vi "DBM_GetTimesRange.vi"(8 "error in (no error)":errorcluster, 9 "End time":timestamp, 10 "Start time":timestamp, 11 "DBManager in":refnum<class "DBManager.lvclass">) -> (0 "error out":errorcluster, 2 "Work period":T1[](array[typedef]), 3 "DBManager out":refnum<class "DBManager.lvclass">)   [LabVIEW 2015, in "DBManager.lvclass"]
uses:
  DBManager.lvclass
  WorkDay.ctl
  DBManager.lvclass/DBManager.ctl
  <vilib>/drjdpowell/SQLite Library/SQL Statement/SQL Statement.lvclass/SQL Statement.ctl
  <vilib>/drjdpowell/SQLite Library/SQL Statement/Column I64.vi
  <vilib>/drjdpowell/SQLite Library/SQL Statement/Bind Timestamp (Real).vi
  <vilib>/drjdpowell/SQLite Library/SQL Statement/Bind Real.vi
  <vilib>/drjdpowell/SQLite Library/SQL Statement/Error Message.vi
  <vilib>/drjdpowell/SQLite Library/SQL Statement/Column Timestamp.vi
  <vilib>/drjdpowell/SQLite Library/SQL Statement/SQL Statement.lvclass
  <vilib>/drjdpowell/SQLite Library/SQL Connection/Connection.lvclass
panel:
  # "Connector Pane"
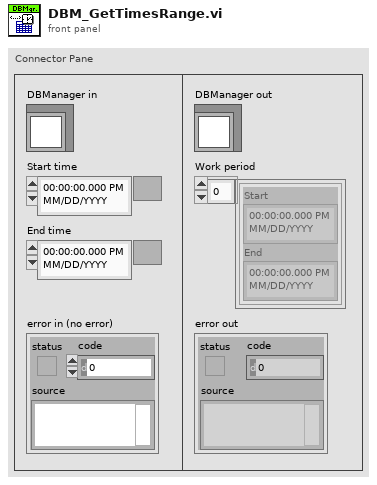
[diagram p1: front panel]
types:
  T1 = typedef "WorkDay.ctl" = cluster{"Start":timestamp, "End":timestamp}
  T2 = cluster{"Previus":timestamp, "Column:Get Column Timestamp":timestamp}[]
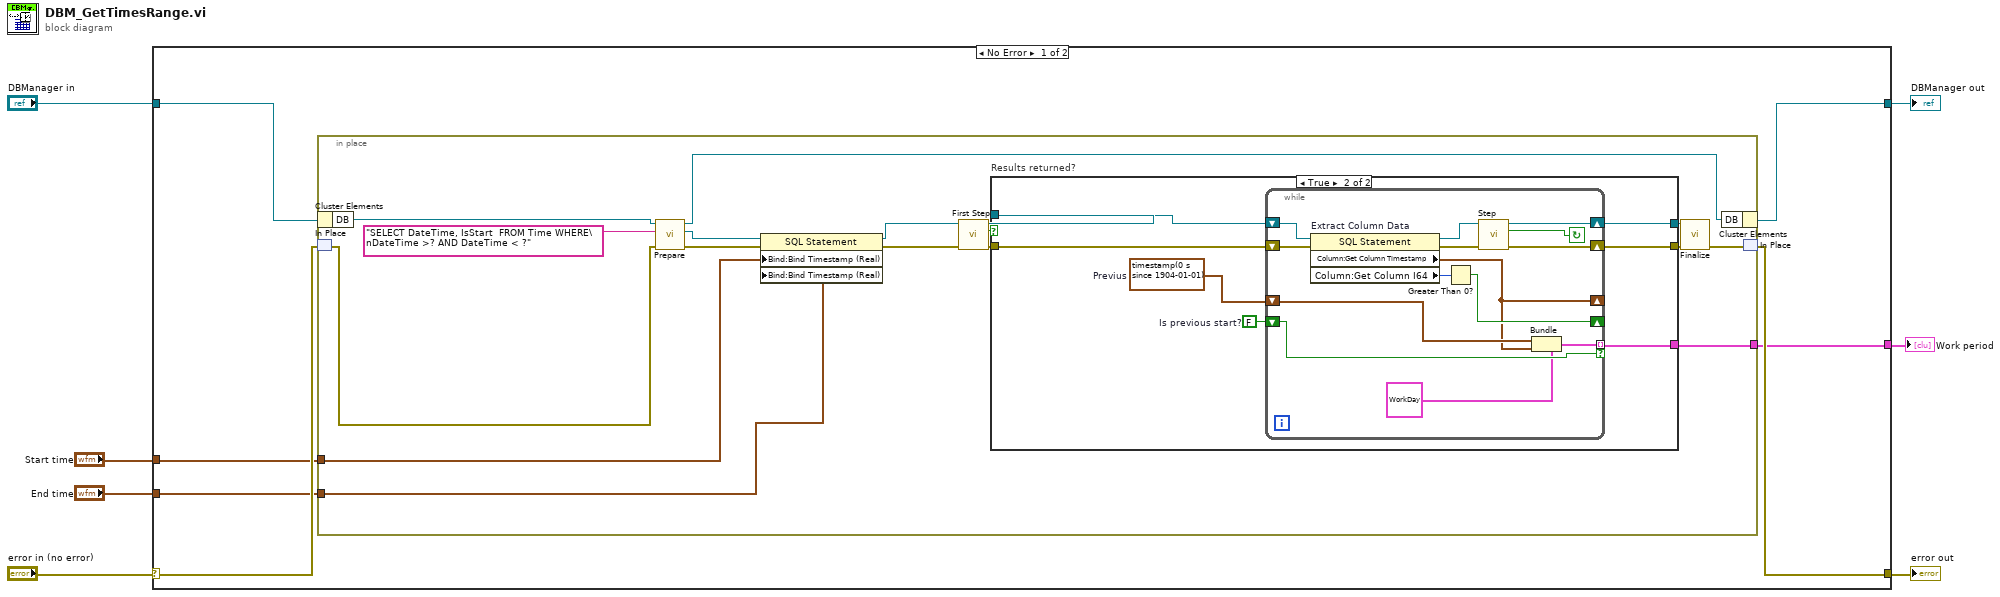
[diagram p0: block diagram]
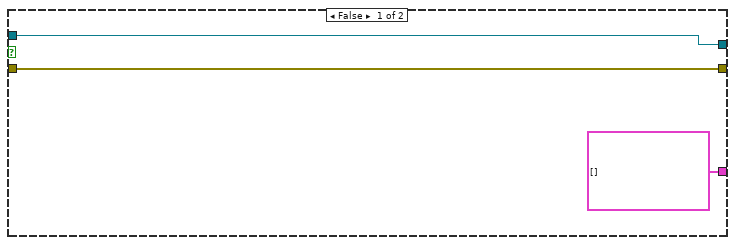
[diagram p2: hidden frame]
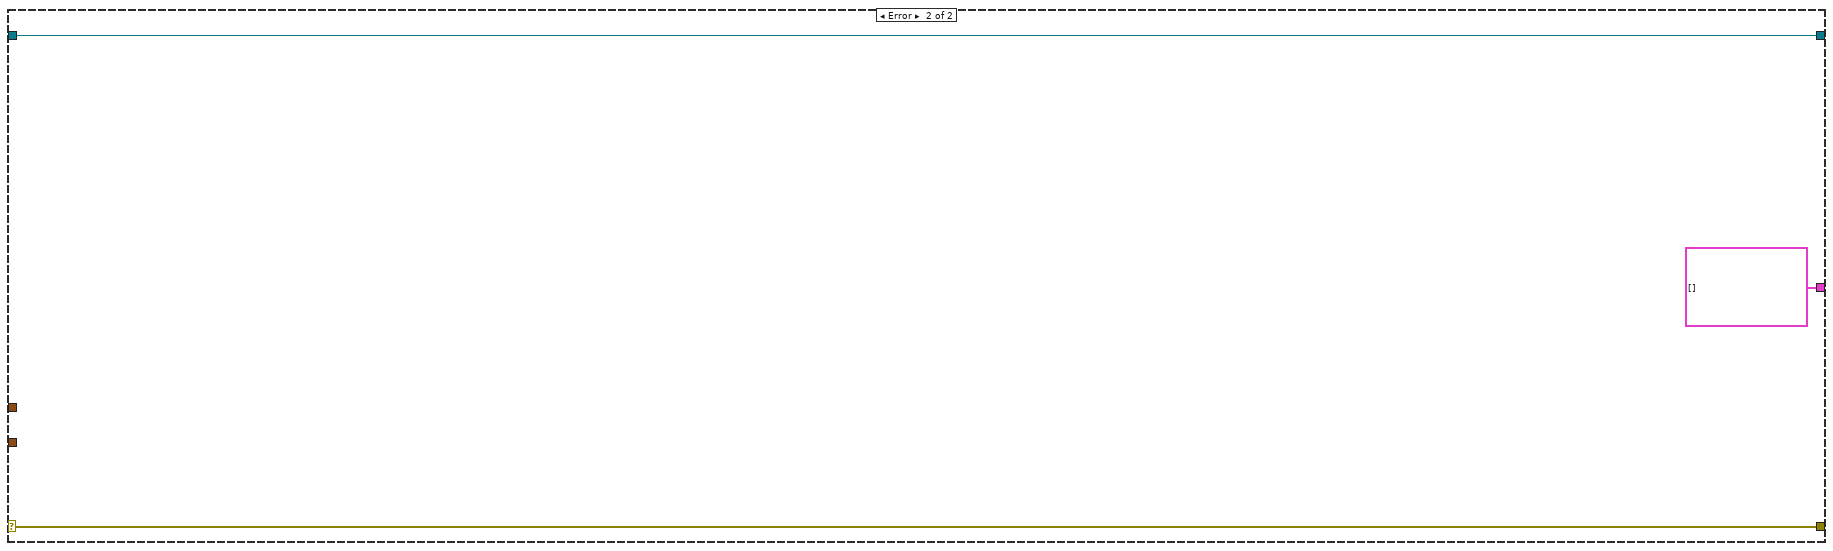
[diagram p3: hidden frame]
diagram:
  n1 = case shown="No Error" "error in (no error)" {
    selector: "error in (no error)" -> [w14 w58]
    tunnel: [w11 w58] -> w6
    tunnel: [w12 w57] -> w4
    tunnel: "DBManager in" -> [w13 w57]
    tunnel: "Start time" -> [w10 _]
    tunnel: "End time" -> [w9 _]
    tunnel: [w8 T2 []] -> w1
    frame No Error {
      n2 = in-place {
        in-place-border: w10 -> [w18]
        in-place-border: w9 -> [w17]
        in-place-border: [w15] -> w8
        n3 = in-place-cluster #1(w13) -> ("DB"=w23:refnum<class "Connection.lvclass">)
        n4 = in-place-match #2(w14) -> (w16:errorcluster)
        n5 = call <vilib>:"Prepare.vi"("error in (no error)"=w16, "SQL"="SELECT DateTime, IsStart  FROM Time WHERE\nDateTime >? AND DateTime < ?" ("SELECT  statement"), "SQLite Connection in"=w23) -> ("error out"=w28:errorcluster, "SQL Statement out"=w20:refnum<class "SQL Statement.lvclass">, "SQLite Connection out"=w24:refnum<class "Connection.lvclass">)  [unwired: 4 in, 2 out]
        n6 = property class="SQL Statement"(reference=w20, error in=w28, "Bind:Bind Timestamp (Real)"=w18, "Bind:Bind Timestamp (Real)"=w17) -> (reference out=w19:refnum<class "SQL Statement.lvclass">, error out=w21:errorcluster)
        n7 = call <vilib>:"First Step.vi"("error in (no error)"=w21, "SQL Statement in"=w19) -> ("error out"=w30:errorcluster, "Row returned"=w31:bool, "SQL Statement out"=w29:refnum<class "SQL Statement.lvclass">)  [unwired: 7 in]
        n8 = case "Results returned?" shown="True" w31 {
          tunnel: [w34 w41] -> w27
          tunnel: [w33 w40] -> w26
          tunnel: w29 -> [w34 w39]
          tunnel: w30 -> [w33 w38]
          tunnel: [T2 [] w35] -> w15
          frame False {
          }
          frame True {
            w36 = FALSE  # Is previous start?
            w37 = timestamp(0 s since 1904-01-01)  # Previus
            n9 = while {
              shift-right: [w55] -> w41
              shift-left: w39 -> [w53]
              shift-right: [w54] -> w40
              shift-left: w38 -> [w52]
              shift-right: [w45] -> _
              shift-left: w37 -> [w46]
              shift-right: [w47] -> _
              shift-left: w36 -> [w43]
              tunnel: [w44] -> w35 mode=indexing if=w43
              stop <- w49 continue-if-true
              n10 = property on="Extract Column Data" class="SQL Statement"(reference=w53, error in=w52) -> (reference out=w51:refnum<class "SQL Statement.lvclass">, error out=w50:errorcluster, "Column:Get Column Timestamp"=w45:timestamp, "Column:Get Column I64"=w48:i64)
              n11 = Greater Than 0?(x=w48) -> (x > 0?=w47:bool)
              n12 = call <vilib>:"Step.vi"("error in (no error)"=w50, "SQL Statement in"=w51) -> ("error out"=w54:errorcluster, "Row returned"=w49:bool, "SQL Statement out"=w55:refnum<class "SQL Statement.lvclass">)  [unwired: 7 in]
              n13 = Bundle(cluster=T1 {"Start"=timestamp(3562905052.3950086 s since 1904-01-01), "End"=timestamp(3562905656.2919016 s since 1904-01-01)} ("WorkDay"), "Start"=w46, "End"=w45) -> (w44:T1)
            }
          }
        }
        n14 = call <vilib>:"Finalize.vi"("error in (no error)"=w26, "SQL Statement in"=w27) -> ("error out"=w25:errorcluster)  [unwired: 9 in]
        n15 = in-place-cluster #1("DB"=w24) -> (w12:refnum<class "DBManager.lvclass">)
        n16 = in-place-match #2(w25) -> (w11:errorcluster)
      }
    }
    frame Error {
    }
  }
  "error out" <- w6
  "DBManager out" <- w4
  "Work period" <- w1
